vi "Program_Active_server.vi"(0 "Client Name":string, 1 "Client Messages":string, 2 "Traverse level State":T1, 3 "Mode":enum16{"Program Active", "Traverse Level State"}(ring), 4 "People to Email":string[](array[string]), 8 "Time till next contact (Sec)":dbl format="%.2f") -> ()   [LabVIEW 2010]
uses:
  ADAM Client/Sub VIs/ADAM Controls/Traverse_Level_State.ctl
  ADAM Client/Sub VIs/ADAM Controls/Ch_description_ADAM.ctl
  ADAM Client/Sub VIs/ADAM Controls/Module_type_ADAM.ctl
  ADAM Client/Sub VIs/ADAM Controls/Function_ADAM.ctl
  ADAM Client/Sub VIs/ADAM Controls/Channel_State.ctl
  ADAM Client/Sub VIs/ADAM Controls/Calib_type_ADAM.ctl
  ADAM Client/Sub VIs/ADAM Controls/Address.ctl
  ADAM_Global.vi
  Anemometry/Anemometry Sub Vis/Globals/Preference_global.vi
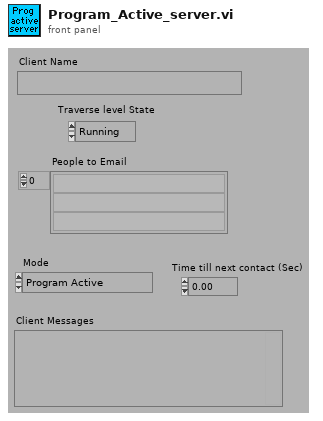
[diagram p1: front panel]
types:
  T1 = typedef "Traverse_Level_State.ctl" = enum16{"Running", "Complete"}
  T2 = typedef "Client_State_Cluster.ctl" = cluster{"Client Name":string, "Traverse level State":T1, "People to Email":string[], "Next Contact Time":dbl}
  T3 = typedef "Ch_description_ADAM.ctl" = cluster{"Ch Name":string, "Type":T4, "Function":T5, "Ch State":T6, "Calibration type":T7, "A":dbl, "B":dbl, "C":dbl, "D":dbl, "Comments":string, "Address":T8, "String":string, "Duty":u16}
  T4 = typedef "Module_type_ADAM.ctl" = enum16{"4011", "4012", "4013", "4014", "4016", "4017", "4018", "4021", "4050", "4052", "4053", "4060", "4080", "5000", "5017", "5018", "5024", "5051", "5056", "5060", "6060", "Tracker", "WEST", "GILL", "JEM", "VICI", "Vaisala", "DRUCK", "Run VI Named:", "IR2100", "PPT", "Comparator", "VIRTUAL", "Hold Value", "Read A", "Read Ch", "Coded", "Client Info", "Web Client", "X10", "Test"}
  T5 = typedef "Function_ADAM.ctl" = enum16{"Analogue Input", "Digital Input", "Event counter", "Event rate", "Analogue Output", "Digital Output", "Relay Output"}
  T6 = typedef "Channel_State.ctl" = enum16{"On", "Off", "Always On", "Always Off"}
  T7 = typedef "Calib_type_ADAM.ctl" = enum16{"Raw", "Bx + A", "Cx^2 + Bx + A", "Dx^3 + Cx^2 + Bx + A", "In Band", "Hi-Tec Q", "Hi-Tec M_dot", "Text"}
  T8 = typedef "Address.ctl" = cluster{"Main":i32, "Ch.":i32, "Sub":i32, "Port Name":string}
  T9 = enum16{"Append to Global", "Read Global then Clear"}
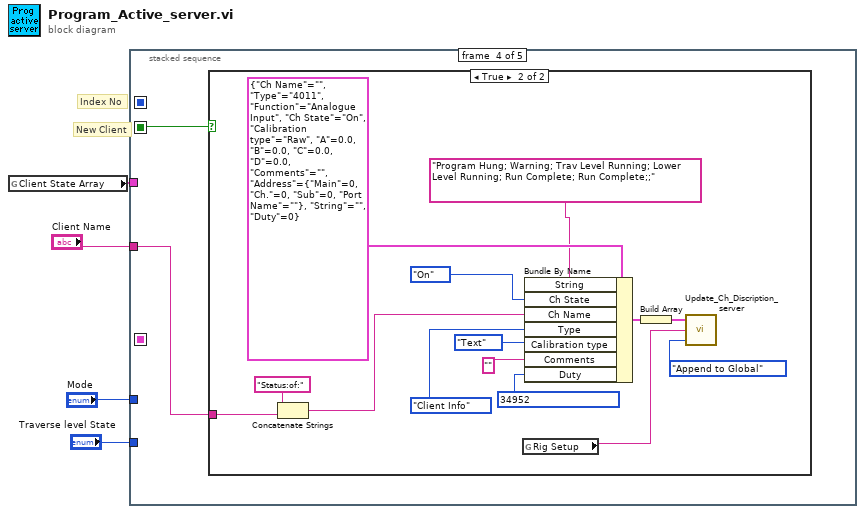
[diagram p0: block diagram]
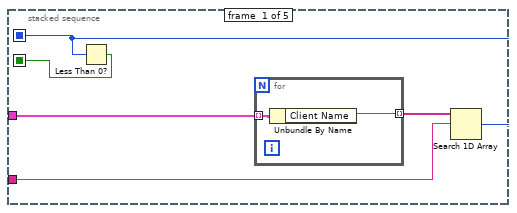
[diagram p2: hidden frame]
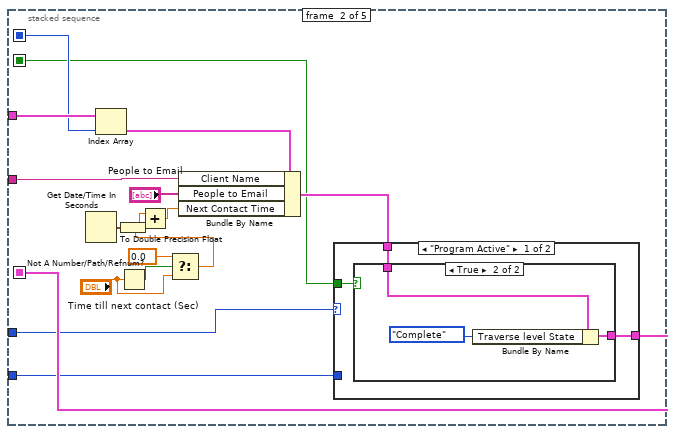
[diagram p3: hidden frame]
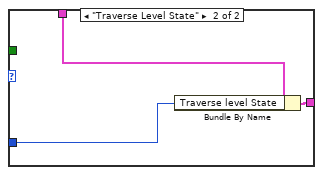
[diagram p5: hidden frame]
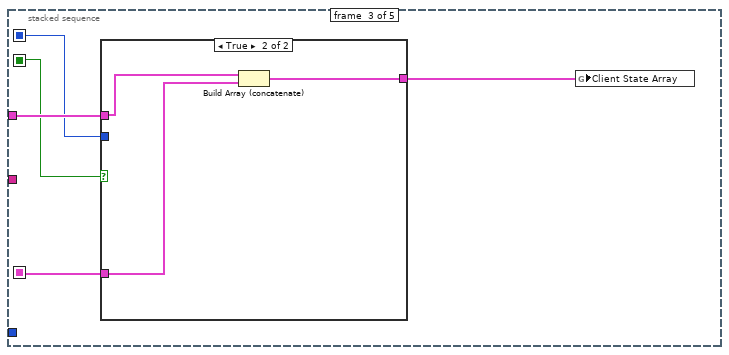
[diagram p6: hidden frame]
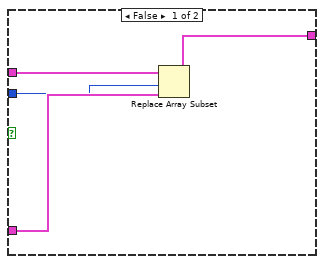
[diagram p7: hidden frame]
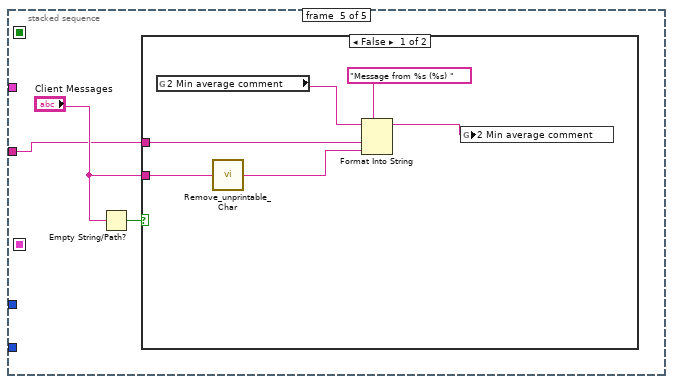
[diagram p9: hidden frame]
diagram:
  # "New Client"
  # "Index No"
  n1 = global read "ADAM_Global.vi" "Client State Array"() -> (w4:T2[])
  n2 = stacked-sequence {
    seq-local: [_ w25 _ _ _] -> [_ _ w42 _ _]
    seq-local: [w7 _ _ _ _] -> [_ w23 w40 _ _]
    seq-local: [w6 _ _ _ _] -> [_ w22 w39 w51 _]
    tunnel: w4 -> [w8 w28 w43 _ _]
    tunnel: "Mode" -> [_ w21 _ _ _]
    tunnel: "Traverse level State" -> [_ w20 _ _ _]
    tunnel: "Client Name" -> [w5 w19 _ w52 w67]
    frame #0 {
      n3 = for {
        tunnel: w8 -> [w11] mode=indexing
        tunnel: [w10] -> w9 mode=indexing
        n4 = Unbundle By Name(w11) -> ("Client Name"=w10:string)
      }
      n5 = Search 1D Array(1D array=w9, element=w5) -> (index of element=w7:i32)  [unwired: 1 out]
      n6 = Less Than 0?(x=w7) -> (x < 0?=w6:bool)
    }
    frame #1 {
      n7 = Get Date/Time In Seconds() -> (seconds since 1Jan1904=w12:timestamp)
      n8 = Index Array(array=w28, index=w23) -> (element=w27:T2)
      n9 = To Double Precision Float(number=w12) -> (double precision float=w18:dbl)
      n10 = Not A Number/Path/Refnum?(number/path/refnum="Time till next contact (Sec)") -> (NaN/Path/Refnum?=w16:bool)
      n11 = Select(t=0.0, s=w16, f="Time till next contact (Sec)") -> (s? t:f=w13:dbl)
      n12 = Add(x=w18, y=w13) -> (x+y=w17:dbl)
      n13 = Bundle By Name(cluster=w27, "Client Name"=w19, "People to Email"="People to Email", "Next Contact Time"=w17) -> (w26:T2)
      n14 = case shown="\"Program Active\"" w21 {
        tunnel: w26 -> [w30 w38]
        tunnel: [w29 w37] -> w25
        tunnel: w22 -> [w31 _]
        tunnel: w20 -> [_ w36]
        frame "Program Active" {
          n15 = case shown="True" w31 {
            tunnel: w30 -> [w32 w35]
            tunnel: [w32 w34] -> w29
            frame False {
            }
            frame True {
              n16 = Bundle By Name(cluster=w35, "Traverse level State"=Traverse_Level_State."Complete" ("Bundle Element")) -> (w34:T2)
            }
          }
        }
        frame "Traverse Level State" {
          n17 = Bundle By Name(cluster=w38, "Traverse level State"=w36) -> (w37:T2)
        }
      }
    }
    frame #2 {
      n18 = case shown="True" w39 {
        tunnel: w43 -> [w47 w48]
        tunnel: w42 -> [w45 w50]
        tunnel: [w46 w49] -> w41
        tunnel: w40 -> [w44 _]
        frame False {
          n19 = Replace Array Subset(array=w47, new element=w45, index=w44) -> (w46:T2[])
        }
        frame True {
          n20 = Build Array (concatenate)(w48, w50) -> (w49:T2[])
        }
      }
      n21 = global write "ADAM_Global.vi" "Client State Array"(w41) -> ()
    }
    frame #3 {
      n22 = case shown="True" w51 {
        tunnel: w52 -> [_ w56]
        frame False {
        }
        frame True {
          n23 = Concatenate Strings("Status:of:", w56) -> (w55:string)
          n24 = global read "Preference_global.vi" "Rig Setup"() -> (w54:string)
          n25 = Bundle By Name(cluster=T3 {"Ch Name"="", "Type"=enum."4011", "Function"=enum."Analogue Input", "Ch State"=enum."On", "Calibration type"=enum."Raw", "A"=0.0, "B"=0.0, "C"=0.0, "D"=0.0, "Comments"="", "Address"={"Main"=0, "Ch."=0, "Sub"=0, "Port Name"=""}, "String"="", "Duty"=0} ("Ch Discription"), "String"="Program Hung; Warning; Trav Level Running; Lower Level Running; Run Complete; Run Complete;;", "Ch State"=Channel_State."On", "Ch Name"=w55, "Type"=Module_type_ADAM."Client Info", "Calibration type"=Calib_type_ADAM."Text", "Comments"="" ("Substring"), "Duty"=u16 34952 ("Bundle Element")) -> (w65:T3)
          n26 = Build Array(w65) -> (w64:T3[])
          n27 = call "Update_Ch_Discription_server.vi"("Mode"=T9."Append to Global", "Client HD name"=w54, "Channels to update In"=w64) -> ()  [unwired: 1 out]
        }
      }
    }
    frame #4 {
      n28 = Empty String/Path?(string/path="Client Messages") -> (empty?=w69:bool)
      n29 = case shown="False" w69 {
        tunnel: "Client Messages" -> [w75 _]
        tunnel: w67 -> [w73 _]
        frame False {
          n30 = global read "ADAM_Global.vi" "2 Min average comment"() -> (w74:string)
          n31 = call "Remove_unprintable_Char.vi"("Input String"=w75) -> ("Output String"=w72:string)
          n32 = Format Into String(format string="Message from %s (%s) ", initial string=w74, w73, w72) -> (resulting string=w70:string)  [unwired: 1 in, 1 out]
          n33 = global write "ADAM_Global.vi" "2 Min average comment"(w70) -> ()
        }
        frame True {
        }
      }
    }
  }
